vi "ImageSimplePixMM (SubVI).vi"(8 "Units":T1(ring), 9 "Pixel resolution":dbl, 10 "Y Array (image frame, pixels)":dbl[](array[numeric]), 11 "X Array (image frame,pixels)":dbl[](array[numeric])) -> (2 "Y Array (image frame, specified units)":dbl[](array[numeric]), 3 "X Array (image frame, specified units)":dbl[](array[numeric]))   [LabVIEW 2016]
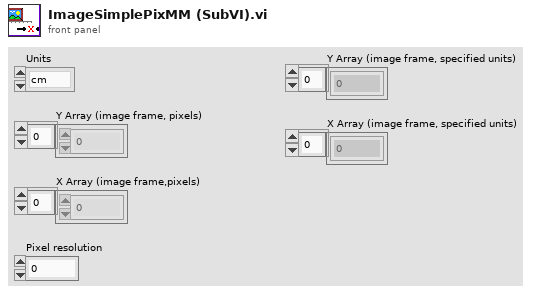
[diagram p1: front panel]
types:
  T1 = enum16{"cm", "mm", "pixels [mm/pix]", "pixels [um/pix]"}
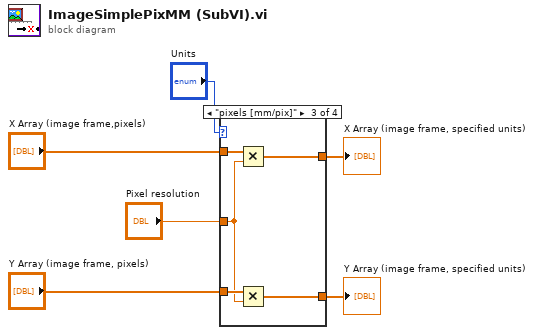
[diagram p0: block diagram]
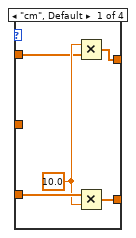
[diagram p2: hidden frame]
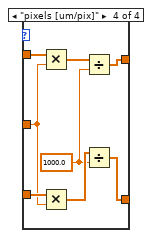
[diagram p4: hidden frame]
diagram:
  n1 = case shown="\"pixels [mm/pix]\"" "Units" {
    tunnel: [w8 w13 w15 w24] -> w3
    tunnel: "Y Array (image frame, pixels)" -> [w11 w13 w16 w25]
    tunnel: "X Array (image frame,pixels)" -> [w9 w12 w18 w23]
    tunnel: [w7 w12 w17 w20] -> w4
    tunnel: "Pixel resolution" -> [_ _ w14 w19]
    frame "cm", Default {
      w10 = 10.0 ("y")
      n2 = Multiply(x=w10, y=w9) -> (x*y=w7:dbl[])
      n3 = Multiply(x=w11, y=w10) -> (x*y=w8:dbl[])
    }
    frame "mm" {
    }
    frame "pixels [mm/pix]" {
      n4 = Multiply(x=w18, y=w14) -> (x*y=w17:dbl[])
      n5 = Multiply(x=w16, y=w14) -> (x*y=w15:dbl[])
    }
    frame "pixels [um/pix]" {
      w21 = 1000.0
      n6 = Multiply(x=w23, y=w19) -> (x*y=w22:dbl[])
      n7 = Multiply(x=w25, y=w19) -> (x*y=w26:dbl[])
      n8 = Divide(x=w22, y=w21) -> (x/y=w20:dbl[])
      n9 = Divide(x=w26, y=w21) -> (x/y=w24:dbl[])
    }
  }
  "X Array (image frame, specified units)" <- w4
  "Y Array (image frame, specified units)" <- w3
